vi "__Init Local List control.vi"(8 "error in (no error)":errorcluster, 11 "FileManager Ctl Refs in":T1) -> (0 "error out":errorcluster, 3 "FileManager Ctl Refs out":T1)   [LabVIEW 2011]
doc: "Initializes the Local list Multicolumn Listbox to a known, default state.\nClears out items and sets column headers to the default values."
uses:
  __File manager Data type.ctl
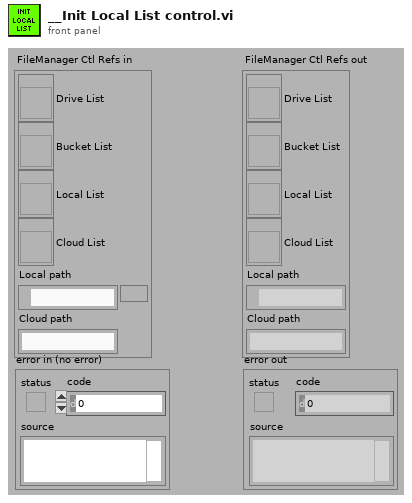
[diagram p1: front panel]
types:
  T1 = typedef "__File manager Data type.ctl" = cluster{"Drive List":refnum<vi>, "Bucket List":refnum<vi>, "Local List":refnum<vi>, "Cloud List":refnum<vi>, "Local path":path, "Cloud path":string}
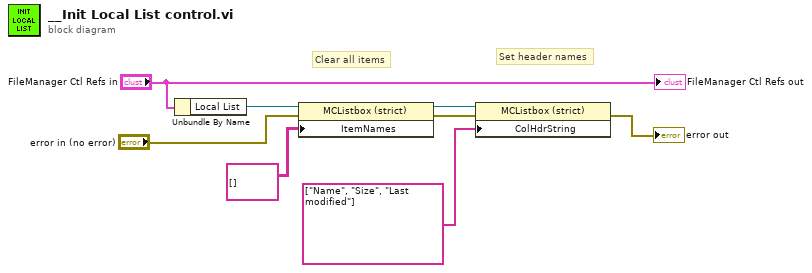
[diagram p0: block diagram]
diagram:
  # "Set header names"
  # "Clear all items"
  n1 = Unbundle By Name("FileManager Ctl Refs in") -> ("Local List"=w2:refnum<vi>)
  n2 = property class="MCListbox (strict)"(reference=w2, error in="error in (no error)", "ItemNames"=string[][] [] ("Item Names")) -> (reference out=w6:refnum<vi>, error out=w7:errorcluster)
  n3 = property class="MCListbox (strict)"(reference=w6, error in=w7, "ColHdrString"=string[] ["Name", "Size", "Last modified"]) -> (error out=→"error out":errorcluster)  [unwired: 1 out]
  "FileManager Ctl Refs out" <- "FileManager Ctl Refs in"
